vi "SetTriggerSource.vi"(8 "Error In":errorcluster, 10 "Trigger Source":T1, 11 "Keithley 6482 In":refnum<visa-resource-name>) -> (0 "Error Out":errorcluster, 3 "Keithley 6482 Out":refnum<visa-resource-name>)   [LabVIEW 2014, in "Keithley-6482-Visa.lvlib"]
uses:
  Keithley-6482-Visa.lvlib
  Controls/TriggerSource.ctl
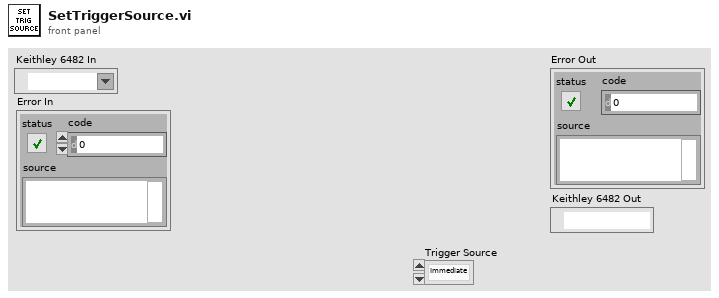
[diagram p1: front panel]
types:
  T1 = typedef "Keithley-6482-Visa.lvlib/TriggerSource.ctl" = enum16{"Immediate", "TLink"}
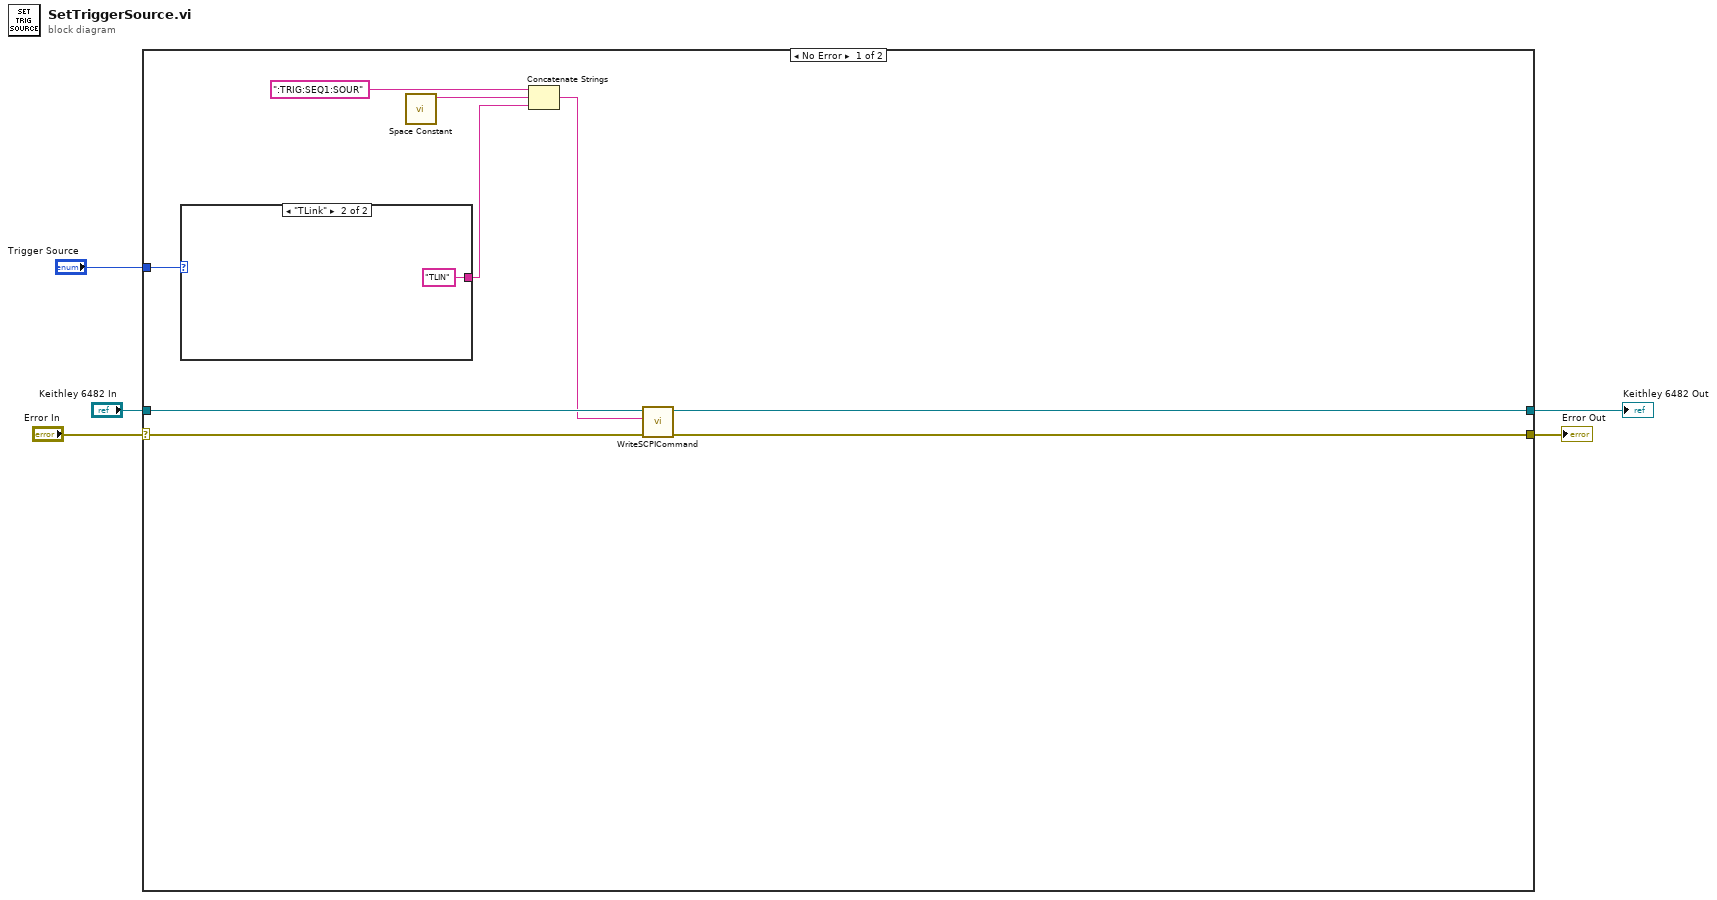
[diagram p0: block diagram]
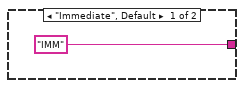
[diagram p2: hidden frame]
diagram:
  n1 = case shown="No Error" "Error In" {
    selector: "Error In" -> [w14 w17]
    tunnel: "Keithley 6482 In" -> [w13 w18]
    tunnel: [w8 w17] -> w3
    tunnel: [w9 w18] -> w2
    tunnel: "Trigger Source" -> [w6 _]
    frame No Error {
      n2 = case shown="\"TLink\"" w6 {
        tunnel: ["IMM" "TLIN"] -> w7
        frame "Immediate", Default {
        }
        frame "TLink" {
        }
      }
      n3 = call <vilib>:"Space Constant.vi"() -> ("String"=w11:string)
      n4 = Concatenate Strings(":TRIG:SEQ1:SOUR" ("string"), w11, w7) -> (w10:string)
      n5 = call "WriteSCPICommand.vi"("Error In"=w14, "SCPI Command"=w10, "Keithley 6482 In"=w13) -> ("Error Out"=w8:errorcluster, "Keithley 6482 Out"=w9:refnum<visa-resource-name>)  [unwired: 7 in]
    }
    frame Error {
    }
  }
  "Error Out" <- w3
  "Keithley 6482 Out" <- w2
